vi "PWM_Lenkung.vi"(0 "vorne rechts":dbl, 1 "vorne links":dbl, 2 "Schräg rechts":dbl, 4 "Schräg links":dbl, 5 "PID gains out 2":T2={"proportional gain (Kc)"=0.5, "integral time (Ti, min)"=1.0, "derivative time (Td, min)"=0.001} {"proportional gain (Kc)" format="%#_10g"; "integral time (Ti, min)" format="%#_10g"; "derivative time (Td, min)" format="%#_10g"}) -> (14 "PWM Lenkung":dbl)   [LabVIEW 2016]
doc: "PID Regelung für Servowert\n05.04.17_Tloe"
uses:
  <vilib>/addons/control/pid/autopid.llb/PID autotuning parameters (adv).ctl
  <vilib>/addons/control/pid/NI_PID_autopid.lvlib
panel:
  out "x-y":dbl format="%.3f"
  in  "konstante":dbl
  in  "multiplikator":dbl
  in  "dt (s)":dbl
  in  "autotuning parameters":T1={"technique"=2, "type of controller"=1, "control specification"=0, "amplitude"=1.0} {"amplitude" format="%.2f"; "control specification" items=["normal", "fast", "slow"]; "type of controller" items=["P", "PI", "PID"]; "technique" items=["Step Open Loop", "Step Closed Loop", "Relay", "PID Relay"]}
  out "Angepasste Werte":T2={"proportional gain (Kc)"=1.0, "integral time (Ti, min)"=0.01, "derivative time (Td, min)"=0.0} {"derivative time (Td, min)" format="%.3f"; "integral time (Ti, min)" format="%.3f"; "proportional gain (Kc)" format="%.3f"}
  out "tuning completed?":bool
  in  "autotune? (F)":bool
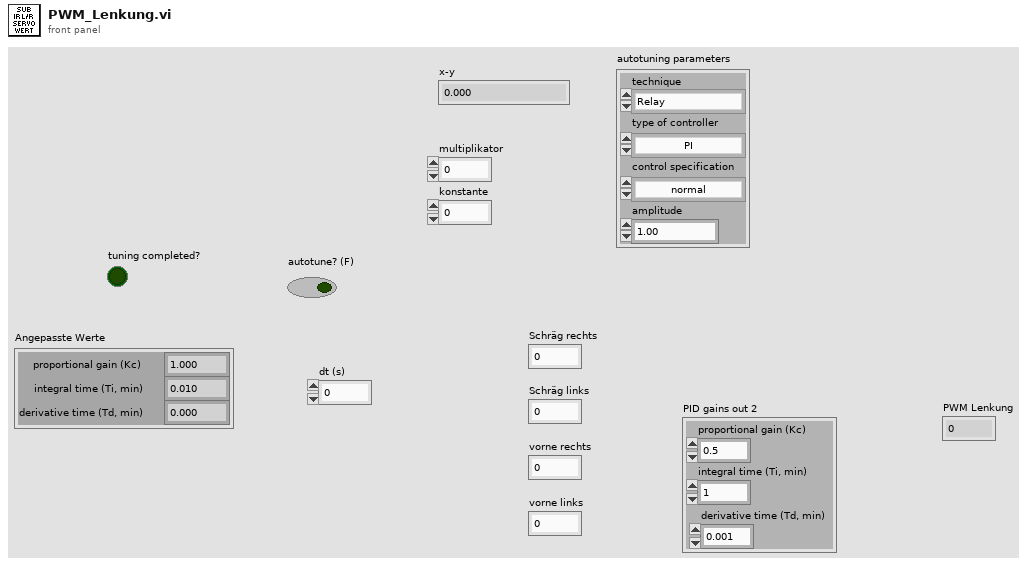
[diagram p1: front panel]
types:
  T1 = typedef "NI_PID_autopid.lvlib/PID autotuning parameters (adv).ctl" = cluster{"technique":u16, "type of controller":u16, "control specification":u16, "amplitude":dbl}
  T2 = cluster{"proportional gain (Kc)":dbl, "integral time (Ti, min)":dbl, "derivative time (Td, min)":dbl}
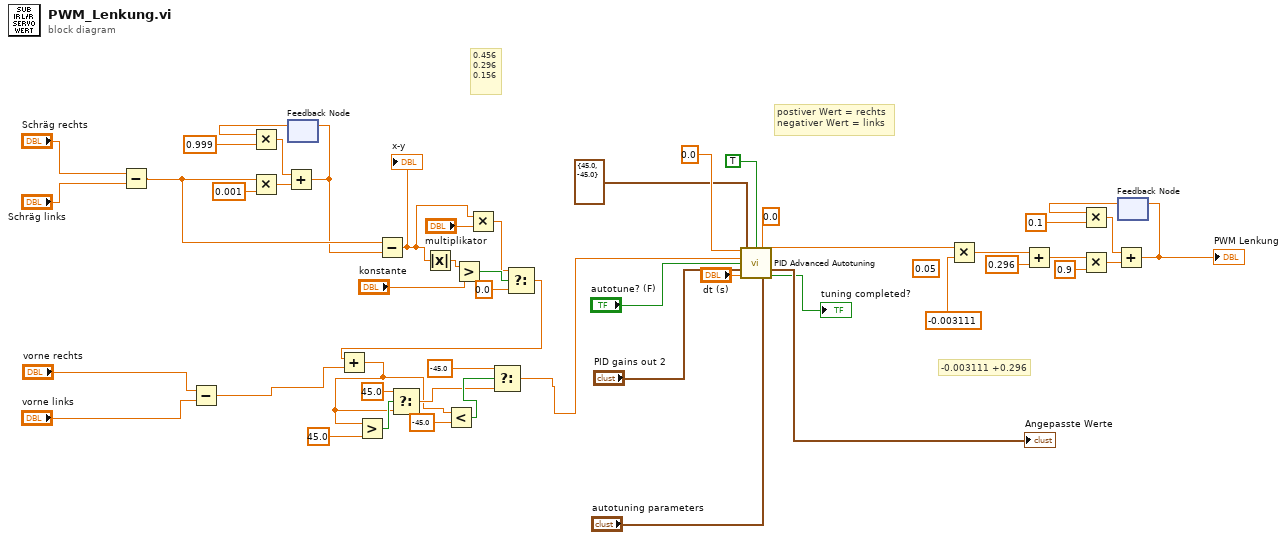
[diagram p0: block diagram]
diagram:
  (unwired) 0.05 ("alpha")
  # "-0.003111 +0.296"
  # "0.456\n0.296\n0.156"
  # "postiver Wert = rechts\nnegativer Wert = links"
  n1 = Subtract(x="Schräg rechts", y="Schräg links") -> (x-y=w20:dbl)
  n2 = Subtract(x="vorne rechts", y="vorne links") -> (x-y=w16:dbl)
  n3 = Multiply(x=w20, y=0.001) -> (x*y=w25:dbl)
  n4 = feedback #1() -> (w21:dbl)  [unwired: 1 in]
  n5 = Multiply(x=w21, y=0.999) -> (x*y=w24:dbl)
  n6 = Add(x=w24, y=w25) -> (x+y=w19:dbl)
  n7 = feedback-in #1(w19) -> ()
  n8 = Subtract(x=w20, y=w19) -> (x-y=w11:dbl)
  "x-y" <- w11
  n9 = Absolute Value(x=w11) -> (abs(x)=w18:dbl)
  n10 = Greater?(x=w18, y="konstante") -> (0:w17:bool)
  n11 = Multiply(x=w11, y="multiplikator") -> (x*y=w13:dbl)
  n12 = Select(t=w13, s=w17, f=0.0) -> (s? t:f=w15:dbl)
  n13 = Add(x=w15, y=w16) -> (x+y=w2:dbl)
  n14 = Greater?(x=w2, y=45.0) -> (0:w9:bool)
  n15 = Select(t=45.0, s=w9, f=w2) -> (s? t:f=w3:dbl)
  n16 = Less?(x=w2, y=-45.0) -> (x < y?=w4:bool)
  n17 = Select(t=-45.0, s=w4, f=w3) -> (s? t:f=w1:dbl)
  n18 = call <vilib>:"PID Advanced Autotuning.vi"("setpoint"=0.0, "output range"=cluster{"output high":dbl, "output low":dbl} {"output high"=45.0, "output low"=-45.0}, "auto? (F)"=TRUE, "manual control"=0.0, "process variable"=w1, "autotune? (F)"="autotune? (F)", "PID gains"="PID gains out 2", "dt (s)"="dt (s)", "autotuning parameters"="autotuning parameters") -> ("output"=w50:dbl, "tuned PID gains"=→"Angepasste Werte":T2, "tuning completed?"=→"tuning completed?":bool)  [unwired: 4 in]
  n19 = Multiply(x=w50, y=-0.003111) -> (x*y=w46:dbl)
  n20 = Add(x=w46, y=0.296) -> (x+y=w48:dbl)
  n21 = Multiply(x=w48, y=0.9) -> (x*y=w44:dbl)
  n22 = feedback #2() -> (w39:dbl)  [unwired: 1 in]
  n23 = Multiply(x=w39, y=0.1) -> (x*y=w43:dbl)
  n24 = Add(x=w43, y=w44) -> (x+y=w40:dbl)
  "PWM Lenkung" <- w40
  n25 = feedback-in #2(w40) -> ()
